vi "Comparision.vi"() -> ()   [LabVIEW 2020]
panel:
  out "In Range?":bool
  out "min(x,y)":dbl
  out "max(x,y)":dbl
  out "Select Output":dbl
  in  "Boolean":bool
  in  "Select Input":dbl
  # "Comparision"
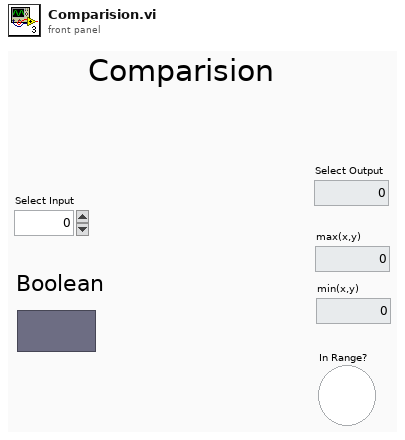
[diagram p1: front panel]
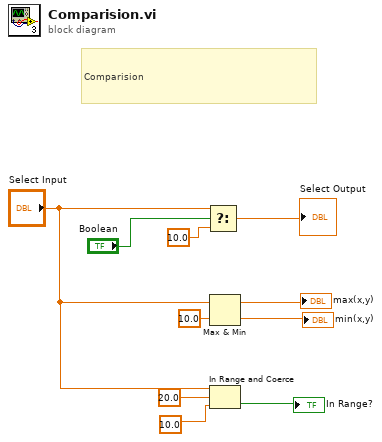
[diagram p0: block diagram]
diagram:
  # "Comparision"
  n1 = Select(t="Select Input", s="Boolean", f=10.0) -> (s? t:f=→"Select Output":dbl)
  n2 = Max & Min(x="Select Input", y=10.0) -> (max(x,y)=→"max(x,y)":dbl, min(x,y)=→"min(x,y)":dbl)
  n3 = In Range and Coerce(upper limit="Select Input", x=20.0, lower limit=10.0) -> (In Range?=→"In Range?":bool)  [unwired: 1 out]
